vi "CAN Jaguar Enable Control.vi"(8 "error in (no error)":errorcluster, 10 "Encoder Initial Position":dbl, 11 "CAN Jaguar Ref":T1={"Device Number"=1, "Control Mode"=enum."Percent VBus", "Inverted"=FALSE, "Semaphore"=refnum, "Max Vout"=12.0, "DevStatus"={"status"=FALSE, "code"=0, "source"=""}}) -> (0 "error out":errorcluster, 3 "CAN Jaguar Ref Out":T1={"Device Number"=0, "Control Mode"=enum."Percent VBus", "Inverted"=FALSE, "Semaphore"=refnum, "Max Vout"=12.0, "DevStatus"={"status"=FALSE, "code"=0, "source"=""}})   [LabVIEW 2009, in "CAN.lvlib"]
uses:
  CAN.lvlib
  SubVIs/CAN Jaguar Ref.ctl
  SubVIs/CAN Jaguar Control Mode.ctl
  SubVIs/CAN Token Message IDs.ctl
panel:
  out "appended array":u8[](array[numeric])
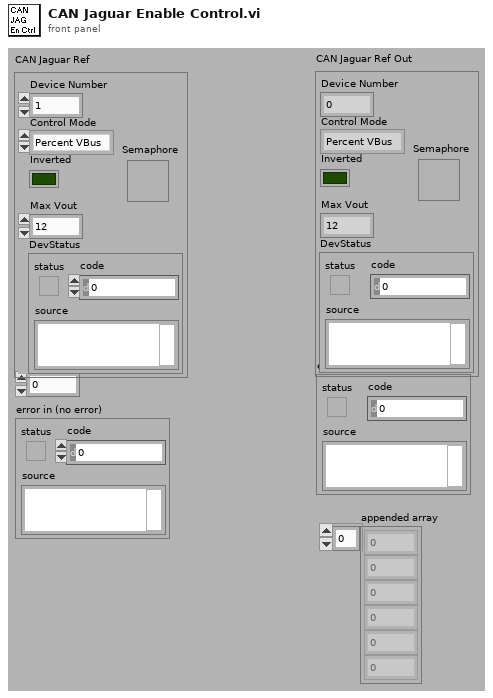
[diagram p1: front panel]
types:
  T1 = typedef "CAN.lvlib/CAN Jaguar Ref.ctl" = cluster{"Device Number":u8, "Control Mode":T2, "Inverted":bool, "Semaphore":T3, "Max Vout":dbl, "DevStatus":errorcluster}
  T2 = typedef "CAN.lvlib/CAN Jaguar Control Mode.ctl" = enum16{"Percent VBus", "Speed", "Position", "Current"}
  T3 = typedef "Semaphore RefNum" = refnum<k1>
  T4 = enum16{"big-endian, network order", "native, host order", "little-endian"}
  T5 = typedef "CAN.lvlib/CAN Token Message IDs.ctl" = u32
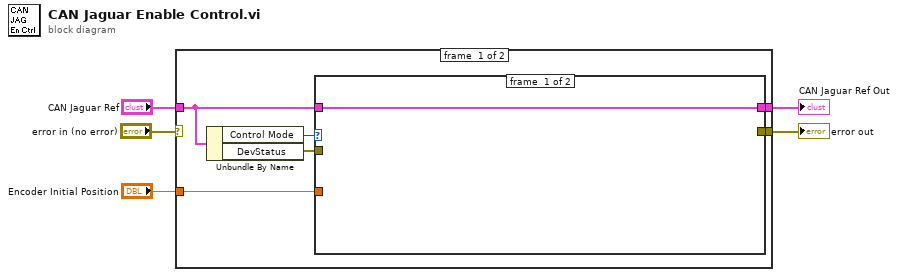
[diagram p0: block diagram]
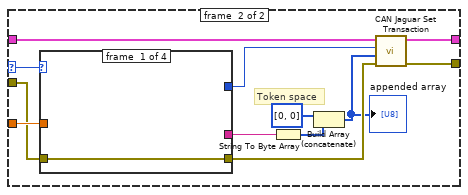
[diagram p2: hidden frame]
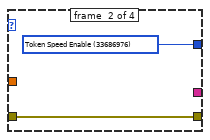
[diagram p3: hidden frame]
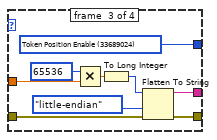
[diagram p4: hidden frame]
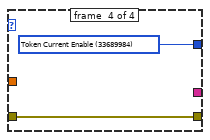
[diagram p5: hidden frame]
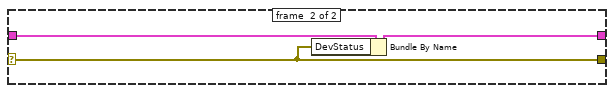
[diagram p6: hidden frame]
diagram:
  n1 = case shown="No Error" "error in (no error)" {
    selector: "error in (no error)" -> [_ w39]
    tunnel: "CAN Jaguar Ref" -> [w9 w41]
    tunnel: [w6 w40] -> w4
    tunnel: [w7 w39] -> w3
    tunnel: "Encoder Initial Position" -> [w11 _]
    frame #0 {
      n2 = Unbundle By Name(w9) -> ("Control Mode"=w10:T2, "DevStatus"=w8:errorcluster)
      n3 = case shown="Default" w10 {
        selector: w10 -> [_ w20]
        tunnel: [w12 w17] -> w6
        tunnel: w9 -> [w12 w18]
        tunnel: w11 -> [_ w24]
        tunnel: w8 -> [_ w19]
        tunnel: [_ w15] -> w7
        frame #0 {
        }
        frame #1 {
          # "Token space"
          n4 = case shown="\"Position\"" w20 {
            tunnel: [_ w27 w36 w38] -> w14
            tunnel: w24 -> [_ _ w35 _]
            tunnel: w19 -> [w25 w26 w32 w37]
            tunnel: [w25 w26 w31 w37] -> w16
            tunnel: [_ _ w28 _] -> w22
            frame #0 {
            }
            frame #1 {
              w27 = T5 33686976 items=["Token Volt Enable"=33685760, "Token Volt Set"=33685824, "Token Speed Enable"=33686976, "Token Speed Set"=33687040, "Token Position Enable"=33689024, "Token Position Set"=33689088, "Token Current Enable"=33689984, "Token Current Set"=33690048] ("CAN Token Message IDs")
            }
            frame #2 {
              w36 = T5 33689024 items=["Token Volt Enable"=33685760, "Token Volt Set"=33685824, "Token Speed Enable"=33686976, "Token Speed Set"=33687040, "Token Position Enable"=33689024, "Token Position Set"=33689088, "Token Current Enable"=33689984, "Token Current Set"=33690048] ("CAN Token Message IDs")
              n5 = Multiply(x=u32 65536, y=w35) -> (x*y=w33:dbl)
              n6 = To Long Integer(number=w33) -> (32bit integer=w29:i32)
              n7 = Flatten To String(anything=w29, byte order (0:big-endian, network order)=T4."little-endian", error in (no error)=w32) -> (data string=w28:string, error out=w31:errorcluster)  [unwired: 1 in, 1 out]
            }
            frame #3 {
              w38 = T5 33689984 items=["Token Volt Enable"=33685760, "Token Volt Set"=33685824, "Token Speed Enable"=33686976, "Token Speed Set"=33687040, "Token Position Enable"=33689024, "Token Position Set"=33689088, "Token Current Enable"=33689984, "Token Current Set"=33690048] ("CAN Token Message IDs")
            }
          }
          n8 = String To Byte Array(string=w22) -> (unsigned byte array=w21:u8[])
          n9 = Build Array (concatenate)(u8[] [0, 0] ("data"), w21) -> (w13:u8[])
          "appended array" <- w13
          n10 = call "CAN Jaguar Set Transaction.vi"("error in"=w16, "Data"=w13, "Message ID"=w14, "CAN Jaguar Ref"=w18) -> ("error out"=w15:errorcluster, "CAN Jaguar Ref Out"=w17:T1)  [unwired: 6 out]
        }
      }
    }
    frame #1 {
      n11 = Bundle By Name(cluster=w41, "DevStatus"=w39) -> (w40:T1)
    }
  }
  "error out" <- w3
  "CAN Jaguar Ref Out" <- w4
